vi "Test set frequency and power.vi"() -> ()   [LabVIEW 2020, in "AM-AM.lvclass"]
uses:
  AM-AM.lvclass
  Instruments/Signal Generator/Signal Generator.lvclass
  AM-AM.lvclass/AM-AM.ctl
panel:
  out "Power":bool[](array[boolean])
  out "Freq":bool[](array[boolean])
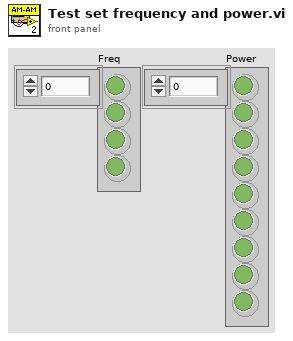
[diagram p1: front panel]
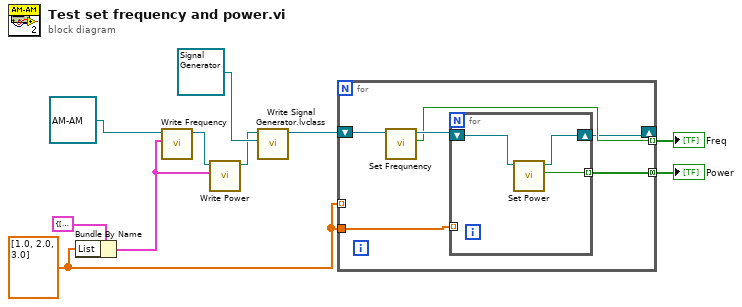
[diagram p0: block diagram]
diagram:
  w5 = dbl[] [1.0, 2.0, 3.0] ("List")
  n1 = Bundle By Name(cluster=cluster{"List":dbl[], "Index":i32, "Last":bool} {"List"=[], "Index"=0, "Last"=FALSE} ("Frequency"), "List"=w5) -> (w1:cluster{"List":dbl[], "Index":i32, "Last":bool})
  n2 = call "Write Frequency.vi"("Frequency"=w1, "AM-AM in"=refnum<class "AM-AM.lvclass"> refnum ("Harmonics.lvclass")) -> ("AM-AM out"=w3:refnum<class "AM-AM.lvclass">)  [unwired: 9 in]
  n3 = call "Write Power.vi"("Power"=w1, "AM-AM in"=w3) -> ("AM-AM out"=w2:refnum<class "AM-AM.lvclass">)  [unwired: 9 in]
  n4 = call "Write Signal Generator.lvclass.vi"("Signal Generator.lvclass"=refnum<class "Signal Generator.lvclass"> refnum, "AM-AM in"=w2) -> ("AM-AM out"=w7:refnum<class "AM-AM.lvclass">)  [unwired: 9 in]
  n5 = for {
    tunnel: [w13] -> w8 mode=indexing
    shift-right: [w11] -> _
    shift-left: w7 -> [w16]
    tunnel: w5 -> [_] mode=indexing
    tunnel: w5 -> [w15]
    tunnel: [w12] -> w4 mode=concatenating
    n6 = call "Set Frequnency.vi"("AM-AM in"=w16) -> ("Last Frequency?"=w13:bool, "AM-AM out"=w14:refnum<class "AM-AM.lvclass">)  [unwired: 7 in, 2 out]
    n7 = for {
      tunnel: w15 -> [_] mode=indexing
      shift-right: [w18] -> w11
      shift-left: w14 -> [w19]
      tunnel: [w17] -> w12 mode=indexing
      n8 = call "Set Power.vi"("AM-AM in"=w19) -> ("Last Power?"=w17:bool, "AM-AM out"=w18:refnum<class "AM-AM.lvclass">)  [unwired: 7 in, 2 out]
    }
  }
  "Freq" <- w8
  "Power" <- w4
